vi "arrayTest.vi"() -> ()   [LabVIEW 2021]
panel:
  out "Y 2":dbl[](array[numeric])
  out "Y":dbl[](array[numeric])
  out "dt":dbl
  out "t0":timestamp
  out "Array 2":dbl[](array[numeric])
  in  "Array":dbl[](array[numeric])
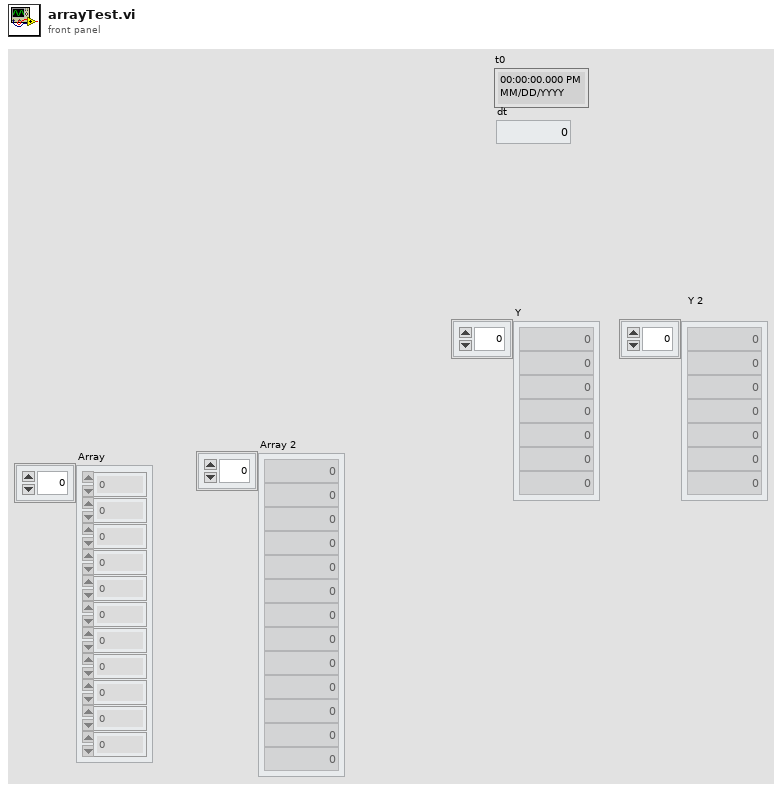
[diagram p1: front panel]
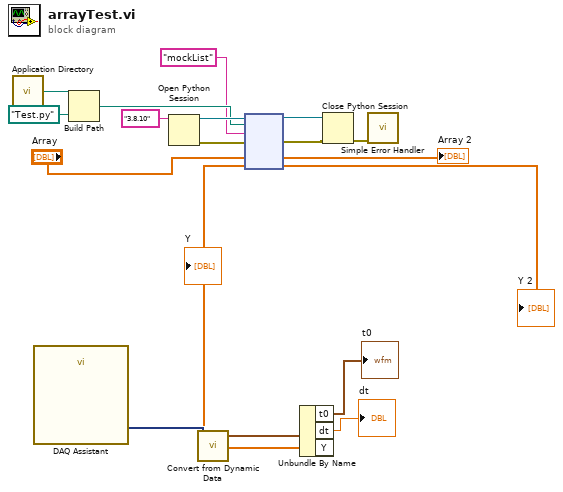
[diagram p0: block diagram]
diagram:
  n1 = call <vilib>:"Application Directory.vi"() -> ("Application Directory"=w13:path)
  n2 = call "DAQ Assistant"() -> ("data"=w6:dynamicdata)  [unwired: 16 in, 3 out]
  n3 = Build Path(base path=w13, name or relative path=path "Test.py") -> (appended path=w11:path)
  n4 = Open Python Session(python version="3.8.10" ("Python version")) -> (session out=w18:refnum<k35>, error out=w17:errorcluster)  [unwired: 2 in]
  n5 = call "Convert from Dynamic Data"("Dynamic Data Type"=w6) -> ("Waveform"=w3:waveform(dbl))  [unwired: 3 in]
  n6 = Unbundle By Name(w3) -> ("t0"=→"t0":timestamp, "dt"=→"dt":dbl, "Y"=w2:dbl[])
  "Y" <- w2
  n7 = node(w18, w11, "mockList" ("function name"), w17, "Array", w2) -> (w15:refnum<k35>, w16:errorcluster, →"Array 2":dbl[], →"Y 2":dbl[])  [unwired: 2 in, 2 out]
  n8 = Close Python Session(session in=w15, error in=w16) -> (11:w9:errorcluster)
  n9 = call <vilib>:"Simple Error Handler.vi"("error in (no error)"=w9) -> ()  [unwired: 4 in, 5 out]
